vi "test_pid.vi"() -> ()   [LabVIEW 2018]
uses:
  <vilib>/addons/control/pid/pid.llb/PID (DBL).vi
  <vilib>/addons/control/pid/NI_PID_pid.lvlib
panel:
  in  "dt (s)":dbl=-1.0 format="%.3f"
  out "Waveform Chart":dbl(graph)
  in  "PID gains":T1={"proportional gain (Kc)"=1.0, "integral time (Ti, min)"=0.01, "derivative time (Td, min)"=0.0} {"derivative time (Td, min)" format="%.3f"; "integral time (Ti, min)" format="%.3f"; "proportional gain (Kc)" format="%.3f"}
  out "output":dbl format="%.2f"
  in  "output range":cluster{"output high":dbl, "output low":dbl}={"output high"=100.0, "output low"=-100.0} {"output low" format="%.2f"; "output high" format="%.2f"}
  in  "stop":bool
  in  "process variable":dbl format="%.2f"
  in  "setpoint":dbl format="%.2f"
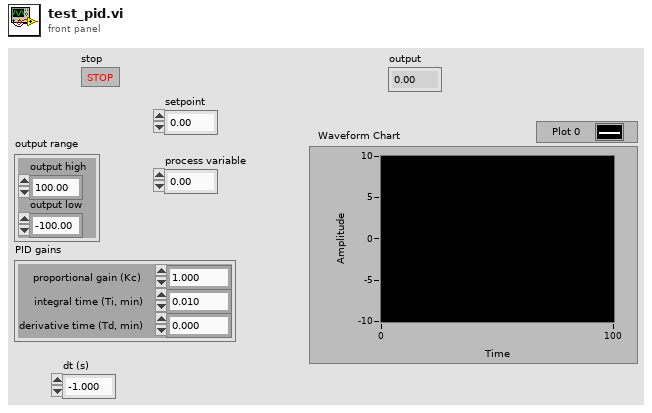
[diagram p1: front panel]
types:
  T1 = cluster{"proportional gain (Kc)":dbl, "integral time (Ti, min)":dbl, "derivative time (Td, min)":dbl}
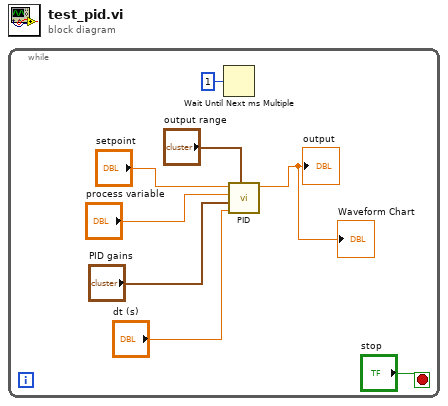
[diagram p0: block diagram]
diagram:
  n1 = while {
    stop <- "stop" stop-if-true
    n2 = Wait Until Next ms Multiple(millisecond multiple=u32 1) -> ()  [unwired: 1 out]
    n3 = call-poly <vilib>:"PID.vi"("output range"="output range", "dt (s)"="dt (s)", "PID gains"="PID gains", "process variable"="process variable", "setpoint"="setpoint") -> ("output"=→"output" →"Waveform Chart":dbl)  [unwired: 5 in, 1 out]
  }
